vi "Splash-Screen.vi"() -> ()   [LabVIEW 2019]
uses:
  Microsoft.Office.Interop.Excel
panel:
  in  "new reference":refnum<k24>
  out "String":string
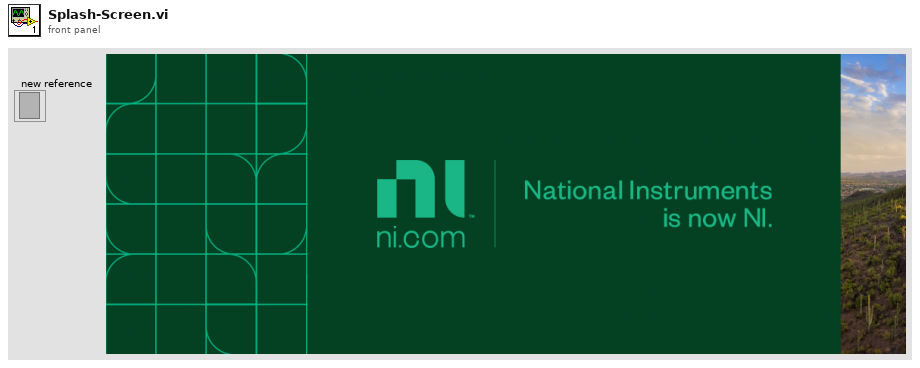
[diagram p1: front panel]
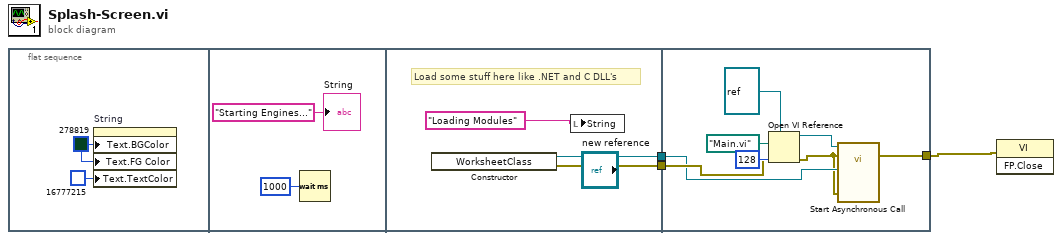
[diagram p0: block diagram]
diagram:
  n1 = flat-sequence {
    tunnel: [w10] -> w3
    tunnel: [w8] -> w2
    tunnel: w3 -> [w13]
    tunnel: w2 -> [w15]
    tunnel: [w11] -> w1
    frame #0 {
      w5 = u32 278819 ("Text.Text Colors:BG Color")
      n2 = property on="String" class="Str"("Text.BGColor"=w5, "Text.FG Color"=w5, "Text.TextColor"=u32 16777215 ("Text.Text Colors:Text Color")) -> ()  [unwired: 2 in, 2 out]
    }
    frame #1 {
      n3 = Wait (ms)(milliseconds to wait=u32 1000) -> ()  [unwired: 1 out]
      "String" <- "Starting Engines..." ("String")
    }
    frame #2 {
      # "Load some stuff here like .NET and C DLL's"
      n4 = constructor class="WorksheetClass"() -> (reference out=w10:refnum<k24>, error out=w8:errorcluster)  [unwired: 3 in, 1 out]
      n5 = local write "String"("Loading Modules" ("String")) -> ()
    }
    frame #3 {
      n6 = Open VI Reference(type specifier VI Refnum (for type only)=refnum<vi> refnum, vi path=path "Main.vi", options=128, error in (no error)=w15) -> (vi reference=w16:refnum<vi>, error out=w12:errorcluster)  [unwired: 2 in]
      n7 = call-by-ref "Start Asynchronous Call"(reference=w16, error in=w12, "Error In"=w12, "new reference"=w13) -> (error out=w11:errorcluster)  [unwired: 10 in, 1 out]
    }
  }
  n8 = invoke class="VI" method="FP.Close"(error in=w1) -> ()  [unwired: 2 in, 3 out]
